vi "Cut merged.vi"(8 "error in (no error)":errorcluster, 11 "Control-Client in":refnum<class "Control-Client.lvclass">) -> (0 "error out":errorcluster, 3 "Control-Client out":refnum<class "Control-Client.lvclass">)   [LabVIEW 2018, in "Control-Client.lvclass"]
uses:
  Control-Client.lvclass
  Experiments/Experiment_merged/Experiment_merged.lvclass
  C:/Users/Sergey Denisov/Documents/REPS/TRANCON/Classes/Experiments/Experiment.lvclass
  Control-Client.lvclass/Control-Client.ctl
  Experiments/Experiment.lvclass
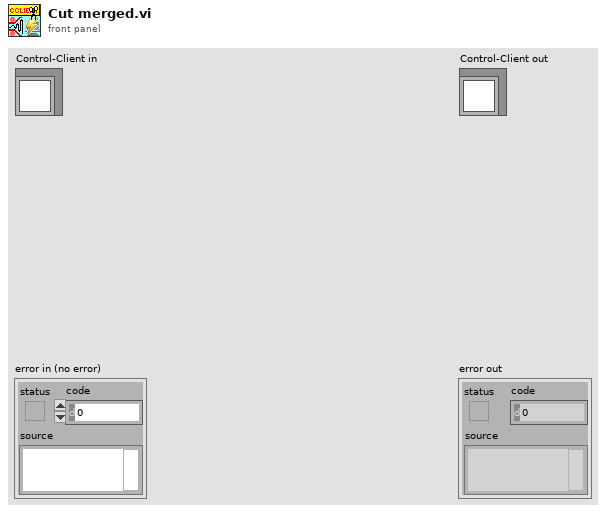
[diagram p1: front panel]
types:
  T1 = cluster{"Max Y pixel":i32, "Min Y pixel":i32, "Max X pixel":i32, "Min X pixel":i32}
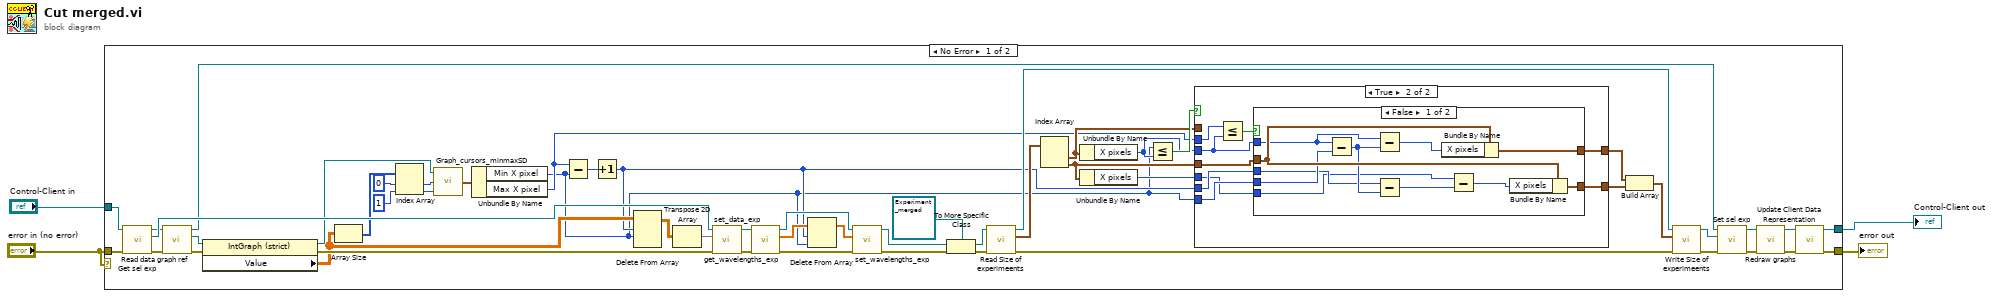
[diagram p0: block diagram]
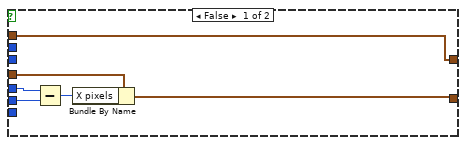
[diagram p2: hidden frame]
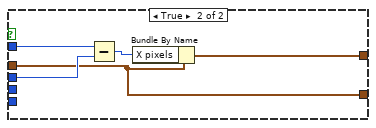
[diagram p3: hidden frame]
diagram:
  n1 = case shown="No Error" "error in (no error)" {
    selector: "error in (no error)" -> [_ w90]
    tunnel: [w57 w90] -> w4
    tunnel: [w56 w89] -> w2
    tunnel: "Control-Client in" -> [w54 w89]
    tunnel: "error in (no error)" -> [w53 _]
    frame No Error {
      n2 = call "Get sel exp.vi"("error in (no error)"=w53, "Control-Client in"=w54) -> ("error out"=w51:errorcluster, "Sel experiment"=w55:refnum<class "Experiment.lvclass">, "Control-Client out"=w52:refnum<class "Control-Client.lvclass">)  [unwired: 7 in]
      n3 = call "Read data graph ref.vi"("error in (no error)"=w51, "Control-Client in"=w52) -> ("error out"=w49:errorcluster, "Exp data graph ref"=w50:refnum<vi>, "Control-Client out"=w45:refnum<class "Control-Client.lvclass">)  [unwired: 7 in]
      n4 = property class="IntGraph (strict)"(reference=w50, error in=w49) -> (reference out=w44:refnum<vi>, error out=w48:errorcluster, "Value"=w32:dbl[][])
      n5 = Array Size(array=w32) -> (size(s)=w43:i32[])
      n6 = Index Array(array=w43, index #1=0 ("index"), index #2=1 ("index")) -> (element #1=w42:i32, element #2=w41:i32)
      n7 = call "Graph_cursors_minmaxSD.vi"("Max Y pixel"=w41, "Max X pixel"=w42, "GRAPH EXPERIMENTAL DATA"=w44) -> ("max/min XY pixels"=w40:T1)
      n8 = Unbundle By Name(w40) -> ("Min X pixel"=w5:i32, "Max X pixel"=w9:i32)
      n9 = Subtract(x=w9, y=w5) -> (x-y=w39:i32)
      n10 = Increment(x=w39) -> (x+1=w7:i32)
      n11 = Delete From Array(array=w32, length=w7, index (row)=w5) -> (array with subset deleted=w31:dbl[][])  [unwired: 1 in, 1 out]
      n12 = Transpose 2D Array(2D array=w31) -> (transposed array=w30:dbl[][])
      n13 = call "set_data_exp.vi"("error in (no error)"=w48, "Data"=w30, "Experiment.lvclass in"=w55) -> ("error out"=w36:errorcluster, "Experiment.lvclass out"=w38:refnum<class "Experiment.lvclass">)  [unwired: 7 in]
      n14 = call "get_wavelengths_exp.vi"("error in (no error)"=w36, "Experiment.lvclass in"=w38) -> ("error out"=w35:errorcluster, "wavelengths"=w34:dbl[], "Experiment.lvclass out"=w37:refnum<class "Experiment.lvclass">)  [unwired: 7 in]
      n15 = Delete From Array(array=w34, length=w7, index=w5) -> (array with subset deleted=w33:dbl[])  [unwired: 1 out]
      n16 = call "set_wavelengths_exp.vi"("error in (no error)"=w35, "wavelengths"=w33, "Experiment.lvclass in"=w37) -> ("error out"=w18:errorcluster, "Experiment.lvclass out"=w24:refnum<class "Experiment.lvclass">)  [unwired: 7 in]
      n17 = To More Specific Class(target class=refnum<class "Experiment_merged.lvclass"> refnum ("Experiment_merged in"), reference=w24, error in=w18) -> (specific class reference=w19:refnum<class "Experiment_merged.lvclass">, error out=w17:errorcluster)
      n18 = call-dynamic "Read Size of experimeents.vi"("error in (no error)"=w17, "Experiment_merged in"=w19) -> ("error out"=w20:errorcluster, "Size of experimeents"=w16:cluster{"X pixels":i32, "Y pixels":i32}[], "Experiment_merged out"=w23:refnum<class "Experiment_merged.lvclass">)  [unwired: 7 in]
      n19 = Index Array(array=w16) -> (element #1=w14:cluster{"X pixels":i32, "Y pixels":i32}, element #2=w13:cluster{"X pixels":i32, "Y pixels":i32})  [unwired: 2 in]
      n20 = Unbundle By Name(w14) -> ("X pixels"=w8:i32)
      n21 = Unbundle By Name(w13) -> ("X pixels"=w6:i32)
      n22 = Less Or Equal?(x=w5, y=w8) -> (x <= y?=w15:bool)
      n23 = case shown="True" w15 {
        tunnel: w6 -> [w63 w64]
        tunnel: w7 -> [w62 w66]
        tunnel: w14 -> [w58 _]
        tunnel: w13 -> [w61 w68]
        tunnel: [w59 w69] -> w12
        tunnel: [w58 w70] -> w11
        tunnel: w9 -> [_ w72]
        tunnel: w8 -> [_ w65]
        tunnel: w5 -> [_ w67]
        frame False {
          n24 = Subtract(x=w63, y=w62) -> (x-y=w60:i32)
          n25 = Bundle By Name(cluster=w61, "X pixels"=w60) -> (w59:cluster{"X pixels":i32, "Y pixels":i32})
        }
        frame True {
          n26 = Less Or Equal?(x=w72, y=w65) -> (x <= y?=w71:bool)
          n27 = case shown="False" w71 {
            tunnel: w65 -> [w78 w88]
            tunnel: w66 -> [w76 w87]
            tunnel: [w81 w85] -> w70
            tunnel: [w82 w84] -> w69
            tunnel: w68 -> [w83 w84]
            tunnel: w67 -> [w80 _]
            tunnel: w64 -> [w74 _]
            frame False {
              n28 = Subtract(x=w78, y=w80) -> (x-y=w77:i32)
              n29 = Subtract(x=w78, y=w77) -> (x-y=w79:i32)
              n30 = Subtract(x=w76, y=w77) -> (x-y=w75:i32)
              n31 = Bundle By Name(cluster=w83, "X pixels"=w79) -> (w81:cluster{"X pixels":i32, "Y pixels":i32})
              n32 = Subtract(x=w74, y=w75) -> (x-y=w73:i32)
              n33 = Bundle By Name(cluster=w83, "X pixels"=w73) -> (w82:cluster{"X pixels":i32, "Y pixels":i32})
            }
            frame True {
              n34 = Subtract(x=w88, y=w87) -> (x-y=w86:i32)
              n35 = Bundle By Name(cluster=w84, "X pixels"=w86) -> (w85:cluster{"X pixels":i32, "Y pixels":i32})
            }
          }
        }
      }
      n36 = Build Array(w11, w12) -> (w10:cluster{"X pixels":i32, "Y pixels":i32}[])
      n37 = call-dynamic "Write Size of experimeents.vi"("error in (no error)"=w20, "Size of experimeents"=w10, "Experiment_merged in"=w23) -> ("error out"=w21:errorcluster, "Experiment_merged out"=w22:refnum<class "Experiment_merged.lvclass">)  [unwired: 7 in]
      n38 = call "Set sel exp.vi"("error in (no error)"=w21, "Experiment"=w22, "Control-Client in"=w45) -> ("error out"=w27:errorcluster, "Control-Client out"=w29:refnum<class "Control-Client.lvclass">)  [unwired: 7 in]
      n39 = call "Redraw graphs.vi"("error in (no error)"=w27, "Control-Client in"=w29) -> ("error out"=w26:errorcluster, "Control-Client out"=w28:refnum<class "Control-Client.lvclass">)  [unwired: 8 in]
      n40 = call "Update Client Data Representation.vi"("error in (no error)"=w26, "Control-Client in"=w28) -> ("error out"=w57:errorcluster, "Control-Client out"=w56:refnum<class "Control-Client.lvclass">)  [unwired: 8 in]
    }
    frame Error {
    }
  }
  "error out" <- w4
  "Control-Client out" <- w2
